vi "ParsePython.vi"(10 "String":string) -> (0 "What is left":string, 1 "functions":string[](array[string]), 2 "Subs":string[](array[string]))   [LabVIEW 2016]
panel:
  in  "functions":u16(ring) items=["Complete Code", "Main Code", "redOnly", "greenOnly", "blueOnly", "allOff", "main"]
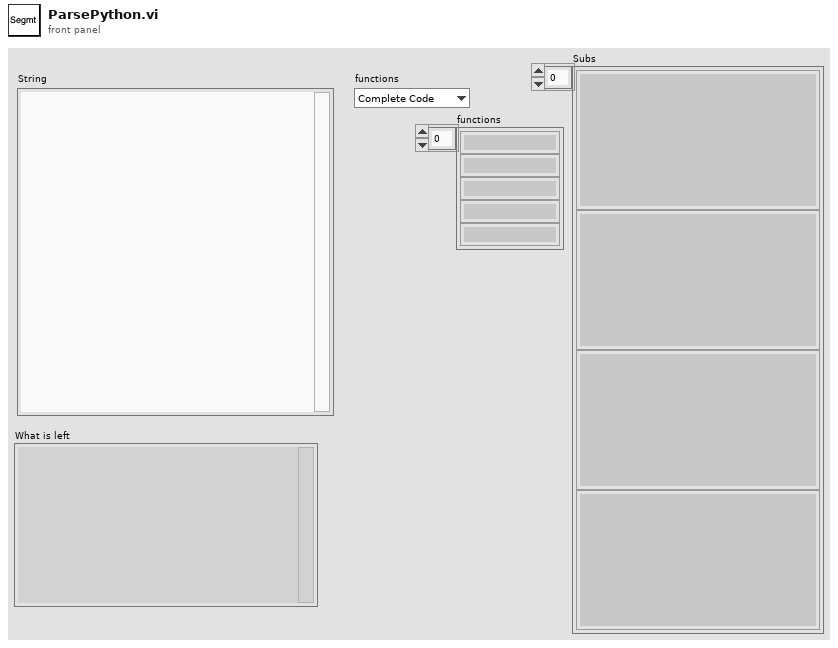
[diagram p1: front panel]
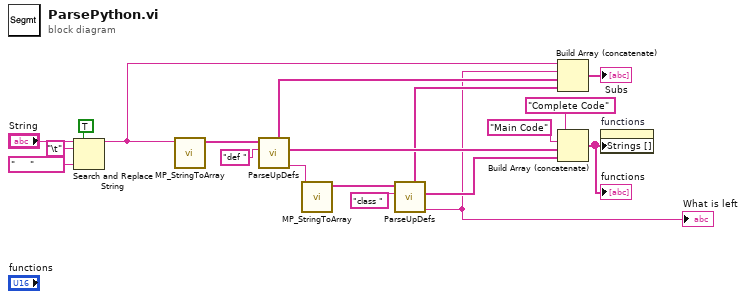
[diagram p0: block diagram]
diagram:
  n1 = Search and Replace String(replace all?=TRUE ("replace all? (F)"), input string="String", search string="\t", replace string="     " ("replace string (\"\")")) -> (result string=w4:string)  [unwired: 4 in, 3 out]
  n2 = call "MP_StringToArray.vi"("write buffer"=w4) -> ("Array"=w19:string[])  [unwired: 10 in]
  n3 = call "ParseUpDefs.vi"("search"="def " ("regular expression"), "Rows"=w19) -> ("left"=w7:string, "Names"=w18:string[], "code"=w10:string[])  [unwired: 7 in]
  n4 = call "MP_StringToArray.vi"("write buffer"=w7) -> ("Array"=w12:string[])  [unwired: 10 in]
  n5 = call "ParseUpDefs.vi"("search"="class " ("regular expression"), "Rows"=w12) -> ("left"=w6:string, "Names"=w11:string[], "code"=w9:string[])  [unwired: 7 in]
  "What is left" <- w6
  n6 = Build Array (concatenate)(w4, w6, w10, w9) -> (→"Subs":string[])
  n7 = Build Array (concatenate)("Complete Code" ("regular expression"), "Main Code" ("regular expression"), w18, w11) -> (w16:string[])
  "functions" <- w16
  n8 = property on="functions" class="Ring (strict)"("Strings []"=w16) -> ()  [unwired: 2 in, 2 out]
